vi "move_to_home_position.vi"(0 "device_index (in) [0=def]":i32, 5 "Error In":errorcluster) -> (19 "Error Out":errorcluster)   [LabVIEW 2013, in "examples.lvlib"]
doc: "Move the motor at the specified index to the home position. Axis may be unwired for single axis controllers.\n\nProduced By:\n\n<B>Kod Integrations, LLC</B>\n4835 Marianne Drive\nMount Airy, MD 21771\nhttp://www.kodintegrations.com\nemail: info@kodintegrations.com\nphone: (240) 687-1288"
uses:
  libraries/examples.lvlib
  classes/Controller/_Controller.lvclass
  common/controls/motor_enabled_state_axes_group.ctl
  libraries/common.lvlib
  common/controls/axis.ctl
  common/controls/linear_direction.ctl
  common/controls/homing_mode.ctl
panel:
  in  "mode (for multi-axis applications only)":T1
  in  "direction":T2
  out "response":string
  out "success?":bool
  in  "axis (def=X)":T3
  in  "clear_buffer? (T)":bool=TRUE
  # "instructions:\n\nAt the specified device index, enter an axis to go-\nto-home and RUN the VI.\n\nNOTE: This example VI makes an attempt to enable\nthe motor at the targeted axis.  If left disabled, the\nmove command will appear to be successful, but\nthe motor physically does not respond."
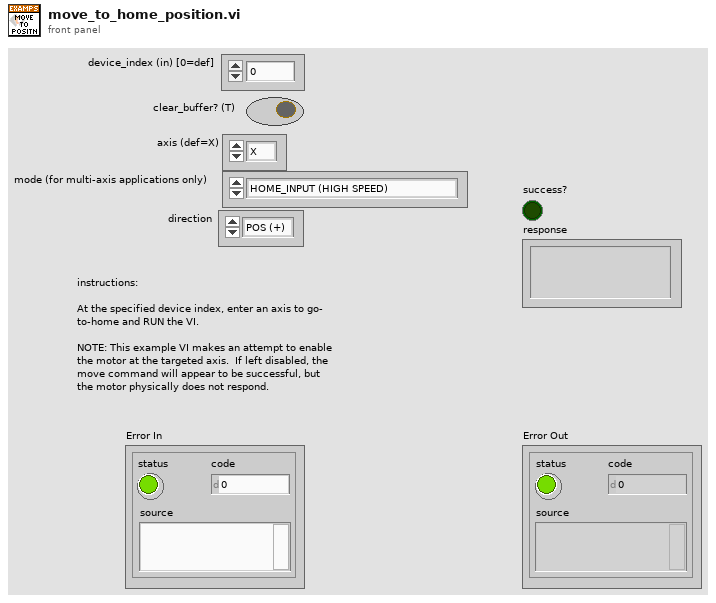
[diagram p1: front panel]
types:
  T1 = typedef "common.lvlib/homing_mode.ctl" = enum16{"HOME_INPUT (HIGH SPEED)", "LIMIT_INPUT", "HOME_INPUT_&_Z-INDEX", "Z-INDEX", "HOME_INPUT (HIGH_&_LOW_SPEED)"}
  T2 = typedef "common.lvlib/linear_direction.ctl" = enum16{"POS (+)", "NEG (-)"}
  T3 = typedef "common.lvlib/axis.ctl" = enum16{"X", "Y", "Z", "U"}
  T4 = typedef "common.lvlib/motor_enabled_state_axes_group.ctl" = cluster{"x-axis":bool, "y-axis":bool, "z-axis":bool, "u-axis":bool}
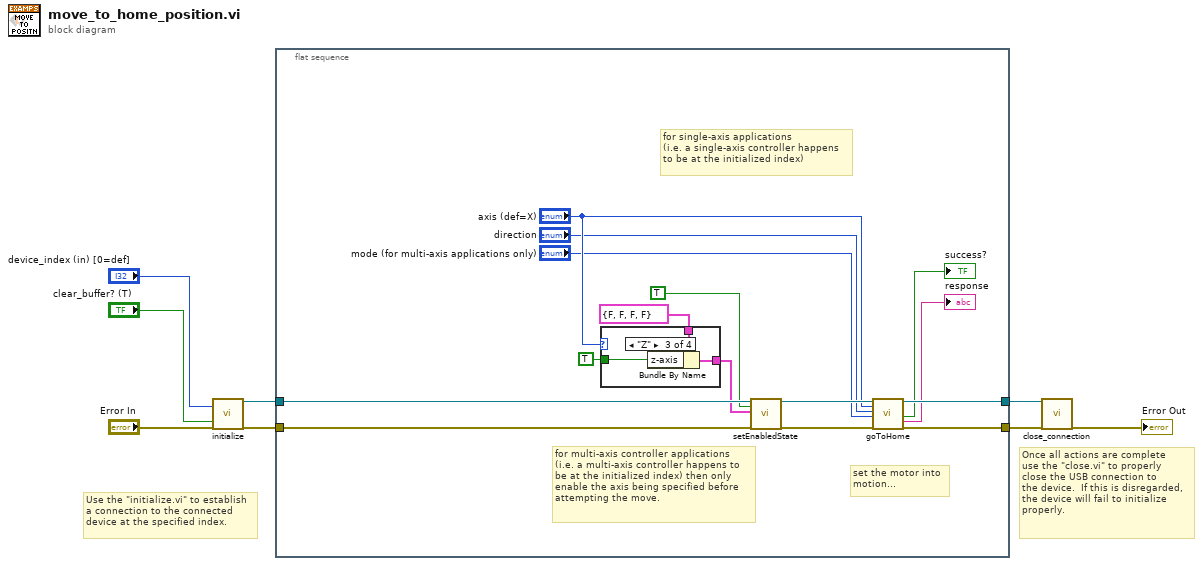
[diagram p0: block diagram]
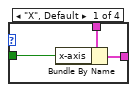
[diagram p2: hidden frame]
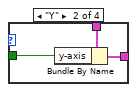
[diagram p3: hidden frame]
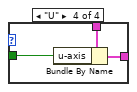
[diagram p4: hidden frame]
diagram:
  # "Once all actions are complete\nuse the \"close.vi\" to properly\nclose the USB connection to \nthe device.  If this is disregarded,\nthe device will fail to initialize \nproperly."
  # "Use the \"initialize.vi\" to establish\na connection to the connected\ndevice at the specified index."
  n1 = call "initialize.vi"("device_index (in) [0=def]"="device_index (in) [0=def]", "clear_buffer? (T)"="clear_buffer? (T)", "error in (no error)"="Error In") -> ("reference (out)"=w5:refnum<class "_Controller.lvclass">, "error out"=w4:errorcluster)  [unwired: 15 in]
  n2 = flat-sequence {
    tunnel: w5 -> [w19]
    tunnel: w4 -> [w18]
    tunnel: [w23] -> w3
    tunnel: [w22] -> w2
    frame #0 {
      # "set the motor into\nmotion..."
      # "for single-axis applications\n(i.e. a single-axis controller happens\nto be at the initialized index)"
      # "for multi-axis controller applications\n(i.e. a multi-axis controller happens to\nbe at the initialized index) then only \nenable the axis being specified before\nattempting the move."
      n3 = case shown="\"Z\"" "axis (def=X)" {
        tunnel: T4 {"x-axis"=FALSE, "y-axis"=FALSE, "z-axis"=FALSE, "u-axis"=FALSE} ("axes_states (for multi-axis applications only)") -> [w26 w29 w32 w35]
        tunnel: [w25 w28 w31 w34] -> w13
        tunnel: TRUE -> [w24 w27 w30 w33]
        frame "X", Default {
          n4 = Bundle By Name(cluster=w26, "x-axis"=w24) -> (w25:T4)
        }
        frame "Y" {
          n5 = Bundle By Name(cluster=w29, "y-axis"=w27) -> (w28:T4)
        }
        frame "Z" {
          n6 = Bundle By Name(cluster=w32, "z-axis"=w30) -> (w31:T4)
        }
        frame "U" {
          n7 = Bundle By Name(cluster=w35, "u-axis"=w33) -> (w34:T4)
        }
      }
      n8 = call-dynamic "setEnabledState.vi"("Controller in"=w19, "state (for single-axis applications only) - (def = DISABLED)"=TRUE ("state (for single-axis applications only)"), "axes_states (for multi-axis applications only) - (def = DISABLED)"=w13, "error in (no error)"=w18) -> ("Controller out"=w17:refnum<class "_Controller.lvclass">, "error out"=w16:errorcluster)  [unwired: 12 in, 2 out]
      n9 = call-dynamic "goToHome.vi"("Controller in"=w17, "axis (for multi-axis applications only)"="axis (def=X)", "dir"="direction", "mode (for multi-axis applications only)"="mode (for multi-axis applications only)", "error in (no error)"=w16) -> ("Controller out"=w23:refnum<class "_Controller.lvclass">, "success?"=→"success?":bool, "response"=→"response":string, "error out"=w22:errorcluster)  [unwired: 11 in]
    }
  }
  n10 = call "close_connection.vi"("reference (in)"=w3, "error in (no error)"=w2) -> ("error out"=→"Error Out":errorcluster)  [unwired: 16 in, 1 out]
